vi "DMSC.start_process.vi"(1 "imageName":string, 2 "argumentString":string, 5 "error in (no error)":errorcluster) -> (19 "error out":errorcluster)   [LabVIEW 2014, in "DMSClient.lvlib"]
doc: "starts a process"
uses:
  DMSClient.lvlib
  DomainManagementUtils/DMSUtils.lvlib
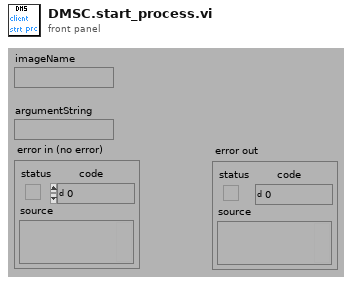
[diagram p1: front panel]
types:
  T1 = enum16{"AddMessage", "AddErrorMessage", "GetMessages"}
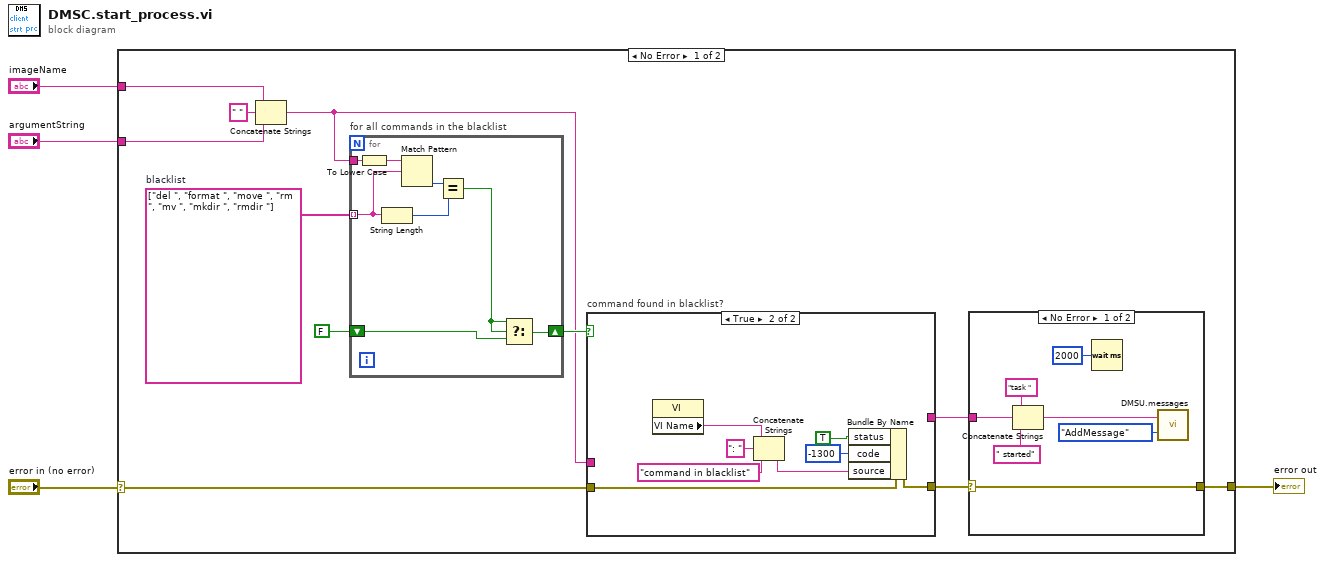
[diagram p0: block diagram]
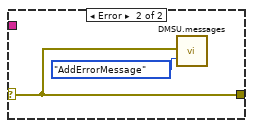
[diagram p2: hidden frame]
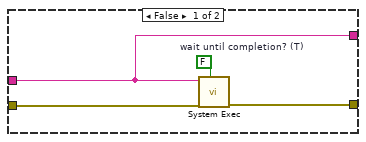
[diagram p3: hidden frame]
diagram:
  n1 = case shown="No Error" "error in (no error)" {
    selector: "error in (no error)" -> [w11 w45]
    tunnel: [w8 w45] -> w4
    tunnel: "imageName" -> [w6 _]
    tunnel: "argumentString" -> [w5 _]
    frame No Error {
      w14 = string[] ["del ", "format ", "move ", "rm ", "mv ", "mkdir ", "rmdir "]  # blacklist
      n2 = Concatenate Strings(w6, " " ("string"), w5) -> (w10:string)
      n3 = for "for all commands in the blacklist" {
        tunnel: w14 -> [w40] mode=indexing
        tunnel: w10 -> [w44]
        shift-right: [w43] -> w12
        shift-left: FALSE -> [w42]
        n4 = To Lower Case(string=w44) -> (all lower case string=w37:string)
        n5 = String Length(string=w40) -> (length=w39:i32)
        n6 = Match Pattern(string=w37, regular expression=w40) -> (offset past match=w41:i32)  [unwired: 1 in, 3 out]
        n7 = Equal?(x=w41, y=w39) -> (x = y?=w38:bool)
        n8 = Select(t=w38, s=w38, f=w42) -> (s? t:f=w43:bool)
      }
      n9 = case "command found in blacklist?" shown="True" w12 {
        tunnel: [w28 w36] -> w9
        tunnel: w11 -> [w27 w33]
        tunnel: w10 -> [w26 _]
        tunnel: [w26 _] -> w7
        frame False {
          w25 = FALSE  # wait until completion? (T)
          n10 = call <vilib>:"System Exec.vi"("wait until completion? (T)"=w25, "error in (no error)"=w27, "command line"=w26) -> ("error out"=w28:errorcluster)  [unwired: 5 in, 3 out]
        }
        frame True {
          n11 = property on="Property Node" class="VI"() -> ("VI Name"=w32:string)  [unwired: 2 in, 2 out]
          n12 = Concatenate Strings(w32, ": " ("string"), "command in blacklist" ("string")) -> (w29:string)
          n13 = Bundle By Name(cluster=w33, "status"=TRUE, "code"=-1300, "source"=w29) -> (w36:errorcluster)
        }
      }
      n14 = case shown="No Error" w9 {
        selector: w9 -> [w18 w23]
        tunnel: [w18 w23] -> w8
        tunnel: w7 -> [w17 _]
        frame No Error {
          n15 = Concatenate Strings("task " ("string"), w17, " started" ("string")) -> (w20:string)
          n16 = Wait (ms)(milliseconds to wait=u32 2000) -> ()  [unwired: 1 out]
          n17 = call "DMSU.messages.vi"("message"=w20, "Action"=T1."AddMessage") -> ()  [unwired: 16 in, 2 out]
        }
        frame Error {
          n18 = call "DMSU.messages.vi"("errorMessage"=w23, "Action"=T1."AddErrorMessage") -> ()  [unwired: 16 in, 2 out]
        }
      }
    }
    frame Error {
    }
  }
  "error out" <- w4
